vi "Get Shutter State.vi"(0 "Notifier Name In":string, 11 "Error In":errorcluster) -> (4 "Notifier Name Out":string, 8 "Shutter State":bool, 15 "Error Out":errorcluster)   [LabVIEW 2020]
uses:
  Microscopes Type Defs/Microscope Notifier.ctl
  Microscopes Type Defs/Microscope Actions.ctl
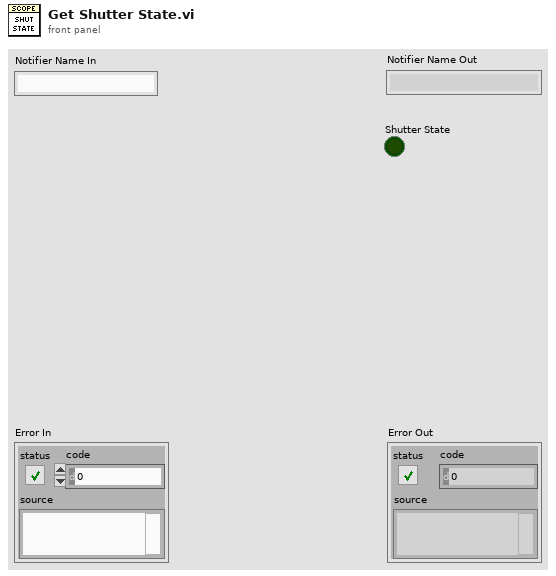
[diagram p1: front panel]
types:
  T1 = typedef "Microscope Notifier.ctl" = cluster{"Actions":T2, "Action Done":bool, "Objective Index":u8, "Objective Z Position (um)":dbl, "Lamp Index":u8, "Lamp State":bool, "Output Port":u8, "Shutter Index":u8, "Shutter State":bool, "Dichroic Wheel Position":u8, "Parameter":string, "Parameter Value":string, "Base Locked?":bool, "Obj Speed":u32, "Obj Acceleration":u32, "Obj Deceleration":u32, "Lamp Power (%)":dbl}
  T2 = typedef "Microscope Actions.ctl" = enum16{"Do Nothing", "Lock Base", "Lock Focus Knob", "Get Objective Index", "Get Objective Z Position", "Get Lamp State", "Get Lamp Power", "Get Output Port", "Get Shutter State", "Get Dichroic Wheel Position", "Set Lamp Index", "Set Shutter Index", "Set Objective Z Position", "Set Lamp State", "Set Lamp Power", "Set Output Port", "Set Shutter State", "Set Dichroic Wheel Position", "Set Objective", "Abort Move", "Set Parameter", "Get Parameter", "Quit"}
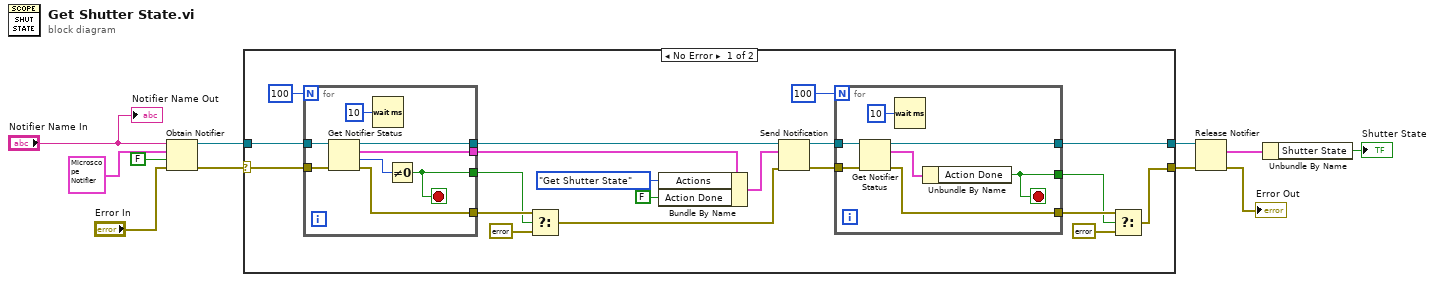
[diagram p0: block diagram]
diagram:
  n1 = Obtain Notifier(name (unnamed)="Notifier Name In", notification data type=T1 {"Actions"=enum."Get Objective Index", "Action Done"=FALSE, "Objective Index"=0, "Objective Z Position (um)"=0.0, "Lamp Index"=0, "Lamp State"=FALSE, "Output Port"=0, "Shutter Index"=0, "Shutter State"=FALSE, "Dichroic Wheel Position"=0, "Parameter"="", "Parameter Value"="", "Base Locked?"=FALSE, "Obj Speed"=0, "Obj Acceleration"=0, "Obj Deceleration"=0, "Lamp Power (%)"=0.0} ("Microscope Notifier"), create if not found? (T)=FALSE, error in (no error)="Error In") -> (notifier out=w8:refnum<notifier>, error out=w9:errorcluster)  [unwired: 1 out]
  n2 = case shown="No Error" w9 {
    selector: w9 -> [w29 w48]
    tunnel: w8 -> [w31 w47]
    tunnel: [w20 w48] -> w4
    tunnel: [w21 w47] -> w5
    frame No Error {
      n3 = for {
        N: 100 -> [_]
        tunnel: w31 -> [w46]
        tunnel: [w44] -> w17
        tunnel: [w42] -> w27
        tunnel: w29 -> [w41]
        tunnel: [w40] -> w18
        tunnel: [w39] -> w28
        stop <- w44 stop-if-true
        n4 = Get Notifier Status(notifier=w46, error in (no error)=w41) -> (notifier out=w42:refnum<notifier>, current notification=w39:T1, # waiting=w45:i32, error out=w40:errorcluster)  [unwired: 1 out]
        n5 = Wait (ms)(milliseconds to wait=u32 10) -> ()  [unwired: 1 out]
        n6 = Not Equal To 0?(x=w45) -> (x != 0?=w44:bool)
      }
      n7 = Select(t=w18, s=w17, f=errorcluster {"status"=TRUE, "code"=0, "source"="IX81 Base Error: Base busy time out."}) -> (s? t:f=w16:errorcluster)
      n8 = Bundle By Name(cluster=w28, "Actions"=Microscope_Actions."Get Shutter State", "Action Done"=FALSE) -> (w26:T1)
      n9 = Send Notification(notification=w26, notifier=w27, error in (no error)=w16) -> (notifier out=w22:refnum<notifier>, error out=w25:errorcluster)
      n10 = for {
        N: 100 -> [_]
        tunnel: w22 -> [w38]
        tunnel: [w36] -> w21
        tunnel: w25 -> [w35]
        tunnel: [w34] -> w14
        tunnel: [w32] -> w13
        stop <- w32 stop-if-true
        n11 = Get Notifier Status(notifier=w38, error in (no error)=w35) -> (notifier out=w36:refnum<notifier>, current notification=w33:T1, error out=w34:errorcluster)  [unwired: 2 out]
        n12 = Wait (ms)(milliseconds to wait=u32 10) -> ()  [unwired: 1 out]
        n13 = Unbundle By Name(w33) -> ("Action Done"=w32:bool)
      }
      n14 = Select(t=w14, s=w13, f=errorcluster {"status"=TRUE, "code"=0, "source"="IX81 Base Error: Action didn't complete."}) -> (s? t:f=w20:errorcluster)
    }
    frame Error {
    }
  }
  n15 = Release Notifier(notifier=w5, error in (no error)=w4) -> (last notification=w2:T1, error out=→"Error Out":errorcluster)  [unwired: 1 in, 1 out]
  n16 = Unbundle By Name(w2) -> ("Shutter State"=→"Shutter State":bool)
  "Notifier Name Out" <- "Notifier Name In"
